vi "Comunicacao_com_LogTcs.vi"   [LabVIEW 2012]
uses:
  Global_Telescopio.vi
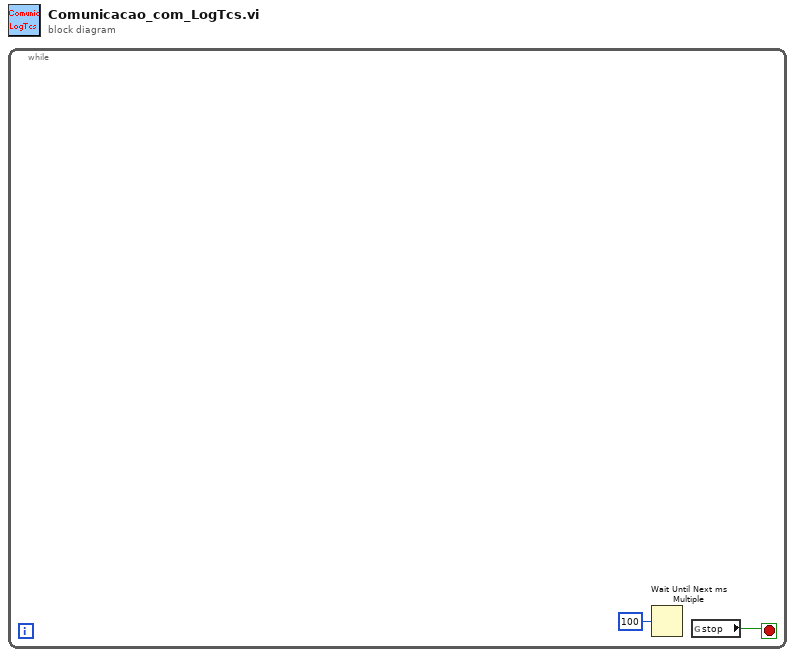
[diagram p0: block diagram]
diagram:
  n1 = while {
    stop <- w2 stop-if-true
    n2 = Wait Until Next ms Multiple(millisecond multiple=u32 100) -> ()  [unwired: 1 out]
    n3 = global read "Global_Telescopio.vi" "stop"() -> (w2:bool)
  }
